vi "PlugIn DS.vi"(6 "String Value":string, 10 "Channel":i32, 11 "Menu":T1=enum."set autonomous") -> ()   [LabVIEW 2019]
uses:
  DS Update Ops.ctl
panel:
  # "Don't place this VI anywhere\nin your API code. It needs to\nbe a dynamically loaded\nwrapper of the main global"
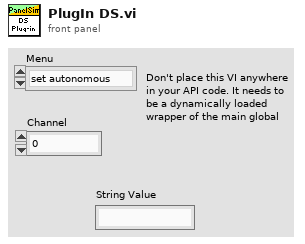
[diagram p1: front panel]
types:
  T1 = typedef "DS Update Ops.ctl" = enum16{"set enabled", "set autonomous", "set test", "set estop", "set fms", "set ds", "set control word", "set match_time", "set station", "set game data", "JSON update", "set name", "get", "transmit initial", "reset"}
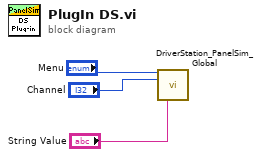
[diagram p0: block diagram]
diagram:
  n1 = call "DriverStation_PanelSim_Global.vi"("menu"="Menu", "Channel"="Channel", "String Value"="String Value") -> ()  [unwired: 11 in, 2 out]
